vi "Connect DSA Master Trigger Routes.vi"(0 "TSM Context":T1, 11 "error in (no error)":errorcluster, 12 "Connect?":bool) -> (15 "error out":errorcluster)   [LabVIEW 2020]
uses:
  <vilib>/NI_TestStand_SemiconductorModule/NI_TestStand_Semiconductor_Module.lvlibp/PinMap/General/SemiconductorModuleContext.ctl
  717ceac2-6976-4702-bc34-c698b76425b4.vi
  <vilib>/NI_TestStand_SemiconductorModule/NI_TestStand_Semiconductor_Module.lvlibp/PinMap/DAQmx/PinToNIDAQmxTask.vi
  <vilib>/NI_TestStand_SemiconductorModule/NI_TestStand_Semiconductor_Module.lvlibp/PinMap/DAQmx/PinToNIDAQmxTasks.vi
  <vilib>/NI_TestStand_SemiconductorModule/NI_TestStand_Semiconductor_Module.lvlibp
  <resource>/objmgr/daqmx.rc
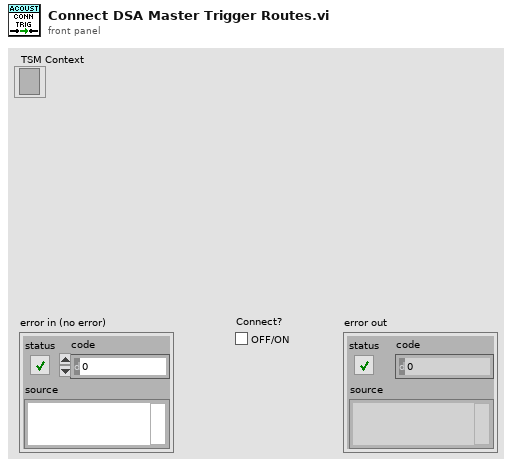
[diagram p1: front panel]
types:
  T1 = typedef "NI_TestStand_Semiconductor_Module.lvlibp/SemiconductorModuleContext.ctl" = refnum<k7>
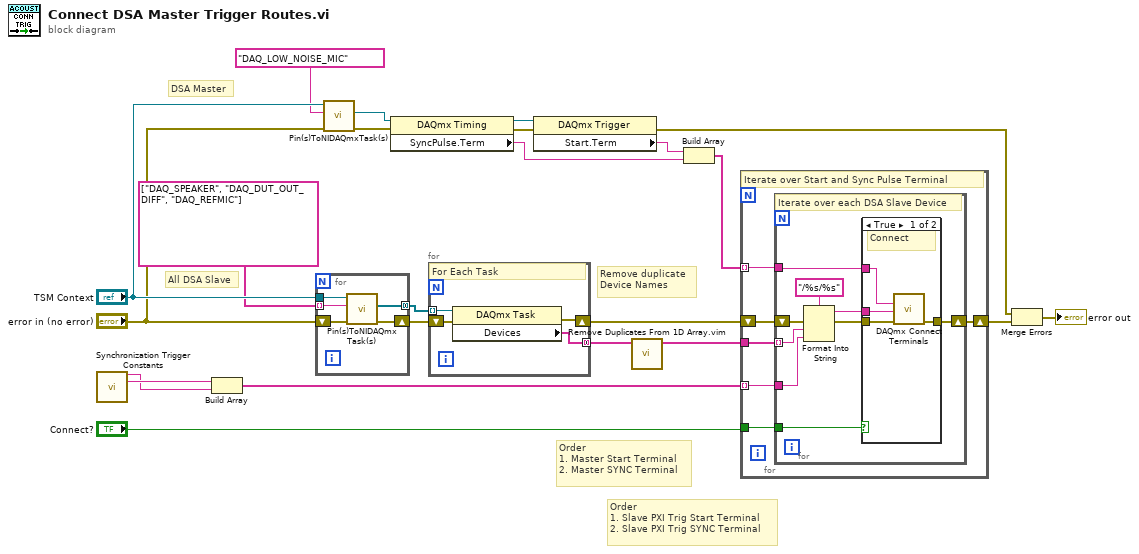
[diagram p0: block diagram]
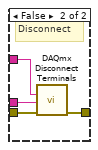
[diagram p2: hidden frame]
diagram:
  # "Order\n1. Slave PXI Trig Start Terminal\n2. Slave PXI Trig SYNC Terminal"
  # "Order\n1. Master Start Terminal\n2. Master SYNC Terminal"
  # "Remove duplicate\nDevice Names"
  # "DSA Master"
  # "All DSA Slave"
  n1 = call "Synchronization Trigger Constants.vi"() -> ("Sync Pulse"=w1:string, "Start Trigger"=w2:string)  [unwired: 13 in, 1 out]
  n2 = Build Array(w2, w1) -> (w19:string[])
  n3 = for {
    tunnel: "TSM Context" -> [w28]
    tunnel: [w27] -> w20 mode=concatenating
    tunnel: tag[] ["DAQ_SPEAKER", "DAQ_DUT_OUT_DIFF", "DAQ_REFMIC"] ("Pins") -> [w26] mode=indexing
    shift-right: [w25] -> w8
    shift-left: "error in (no error)" -> [w24]
    n4 = call-poly <vilib>:"Pin(s)ToNIDAQmxTask(s).vi"("error in (no error)"=w24, "Pin"=w26, "Semiconductor Module Context"=w28) -> ("error out"=w25:errorcluster, "DAQmx Tasks"=w27:refnum<k21>[])  [unwired: 4 in, 3 out]
  }
  n5 = call-poly <vilib>:"Pin(s)ToNIDAQmxTask(s).vi"("error in (no error)"="error in (no error)", "Pin"=tag "DAQ_LOW_NOISE_MIC", "Semiconductor Module Context"="TSM Context") -> ("error out"=w15:errorcluster, "DAQmx Task"=w14:refnum<k21>)  [unwired: 4 in, 3 out]
  n6 = property class="DAQmx Timing"(reference=w14, error in=w15) -> (reference out=w12:refnum<k21>, error out=w13:errorcluster, "SyncPulse.Term"=w16:tag)
  n7 = for {
    tunnel: w20 -> [w32] mode=indexing
    tunnel: [w31] -> w5 mode=concatenating
    shift-right: [w29] -> w6
    shift-left: w8 -> [w30]
    # "For Each Task"
    n8 = property class="DAQmx Task"(reference=w32, error in=w30) -> (error out=w29:errorcluster, "Devices"=w31:tag[])  [unwired: 1 out]
  }
  n9 = property class="DAQmx Trigger"(reference=w12, error in=w13) -> (error out=w10:errorcluster, "Start.Term"=w11:tag)  [unwired: 1 out]
  n10 = call "Remove Duplicates From 1D Array.vim"("array"=w5) -> ("array with duplicates removed"=w4:tag[])  [unwired: 10 in]
  n11 = Build Array(w11, w16) -> (w7:tag[])
  n12 = for {
    tunnel: w4 -> [w38]
    tunnel: w19 -> [w37] mode=indexing
    tunnel: "Connect?" -> [w35]
    tunnel: w7 -> [w34] mode=indexing
    shift-right: [w36] -> w18
    shift-left: w6 -> [w33]
    # "Iterate over Start and Sync Pulse Terminal"
    n13 = for {
      tunnel: w38 -> [w47] mode=indexing
      tunnel: w37 -> [w44]
      tunnel: w35 -> [w42]
      tunnel: w34 -> [w40]
      shift-right: [w43] -> w36
      shift-left: w33 -> [w41]
      # "Iterate over each DSA Slave Device"
      n14 = Format Into String(format string="/%s/%s", error in=w41, w47, w44) -> (resulting string=w45:string, error out=w39:errorcluster)  [unwired: 1 in]
      n15 = case shown="True" w42 {
        tunnel: w45 -> [w51 w55]
        tunnel: [w50 w54] -> w43
        tunnel: w40 -> [w48 w52]
        tunnel: w39 -> [w49 w53]
        frame True {
          # "Connect"
          n16 = call <vilib>:"DAQmx Connect Terminals.vi"("source terminal"=w48, "destination terminal"=w51, "error in"=w49) -> ("error out"=w50:errorcluster)  [unwired: 12 in]
        }
        frame False {
          # "Disconnect"
          n17 = call <vilib>:"DAQmx Disconnect Terminals.vi"("source terminal"=w52, "destination terminal"=w55, "error in"=w53) -> ("error out"=w54:errorcluster)  [unwired: 12 in]
        }
      }
    }
  }
  n18 = Merge Errors(w10, w18) -> (→"error out":errorcluster)
